vi "VITemplate.vi"(8 "Error In":errorcluster, 11 "Data In":T2) -> (0 "Error Out":errorcluster, 3 "Data Out":T2)   [LabVIEW 2019]
doc: "Description of VI"
uses:
  Controls/Data.ctl
  <vilib>/Utility/error.llb/DialogType.ctl
  <vilib>/Utility/miscctls.llb/LVPointTypeDef.ctl
panel:
  out "Control Tab":T1(tab)
  out "Console Out":string
  out "Error Message":string
  out "VI-filename":string
  out "Revision Number":u32
  out "VI Description":string
  out "Callers' Names":string[](array[string])
  out "Code Size":u32
  out "VI Type":T3(ring)
  out "Project name":string
  out "Project filepath":path
  out "VI filepath":path
  out "Project Description":string
  out "VI-Name":string
  # "Common Errors:"
  # "0:"
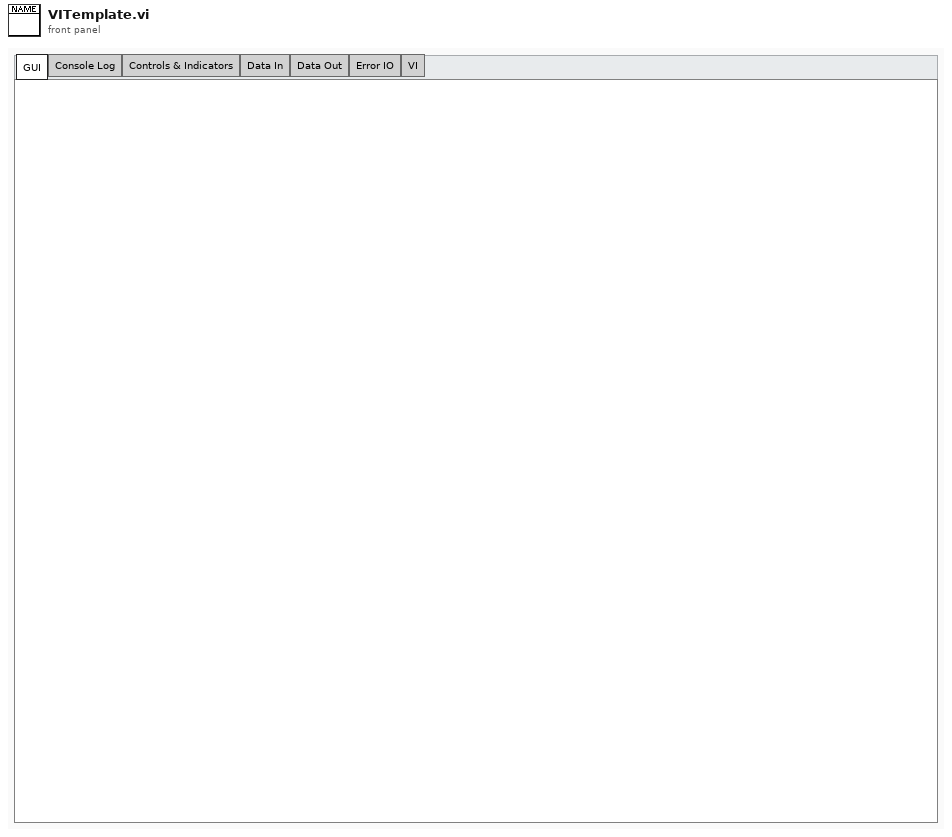
[diagram p1: front panel]
types:
  T1 = enum32{"GUI", "Console Log", "Controls & Indicators", "Data In", "Data Out", "Error IO", "VI"}
  T2 = typedef "Data.ctl" = cluster{"Log":string}
  T3 = enum32{"invalid VI type", "Standard VI", "Control VI", "Global VI", "Polymorphic VI", "Configuration VI", "SubSystem", "Facade VI", "Method VI", "Statechart Diagram VI"}
  T4 = typedef "LVPointTypeDef.ctl" = cluster{"Horizontal":i16, "Vertical":i16}
  T5 = typedef "DialogType.ctl" = u16
  T6 = typedef "LVRectTypeDef.ctl" = cluster{"Left":i16, "Top":i16, "Right":i16, "Bottom":i16}
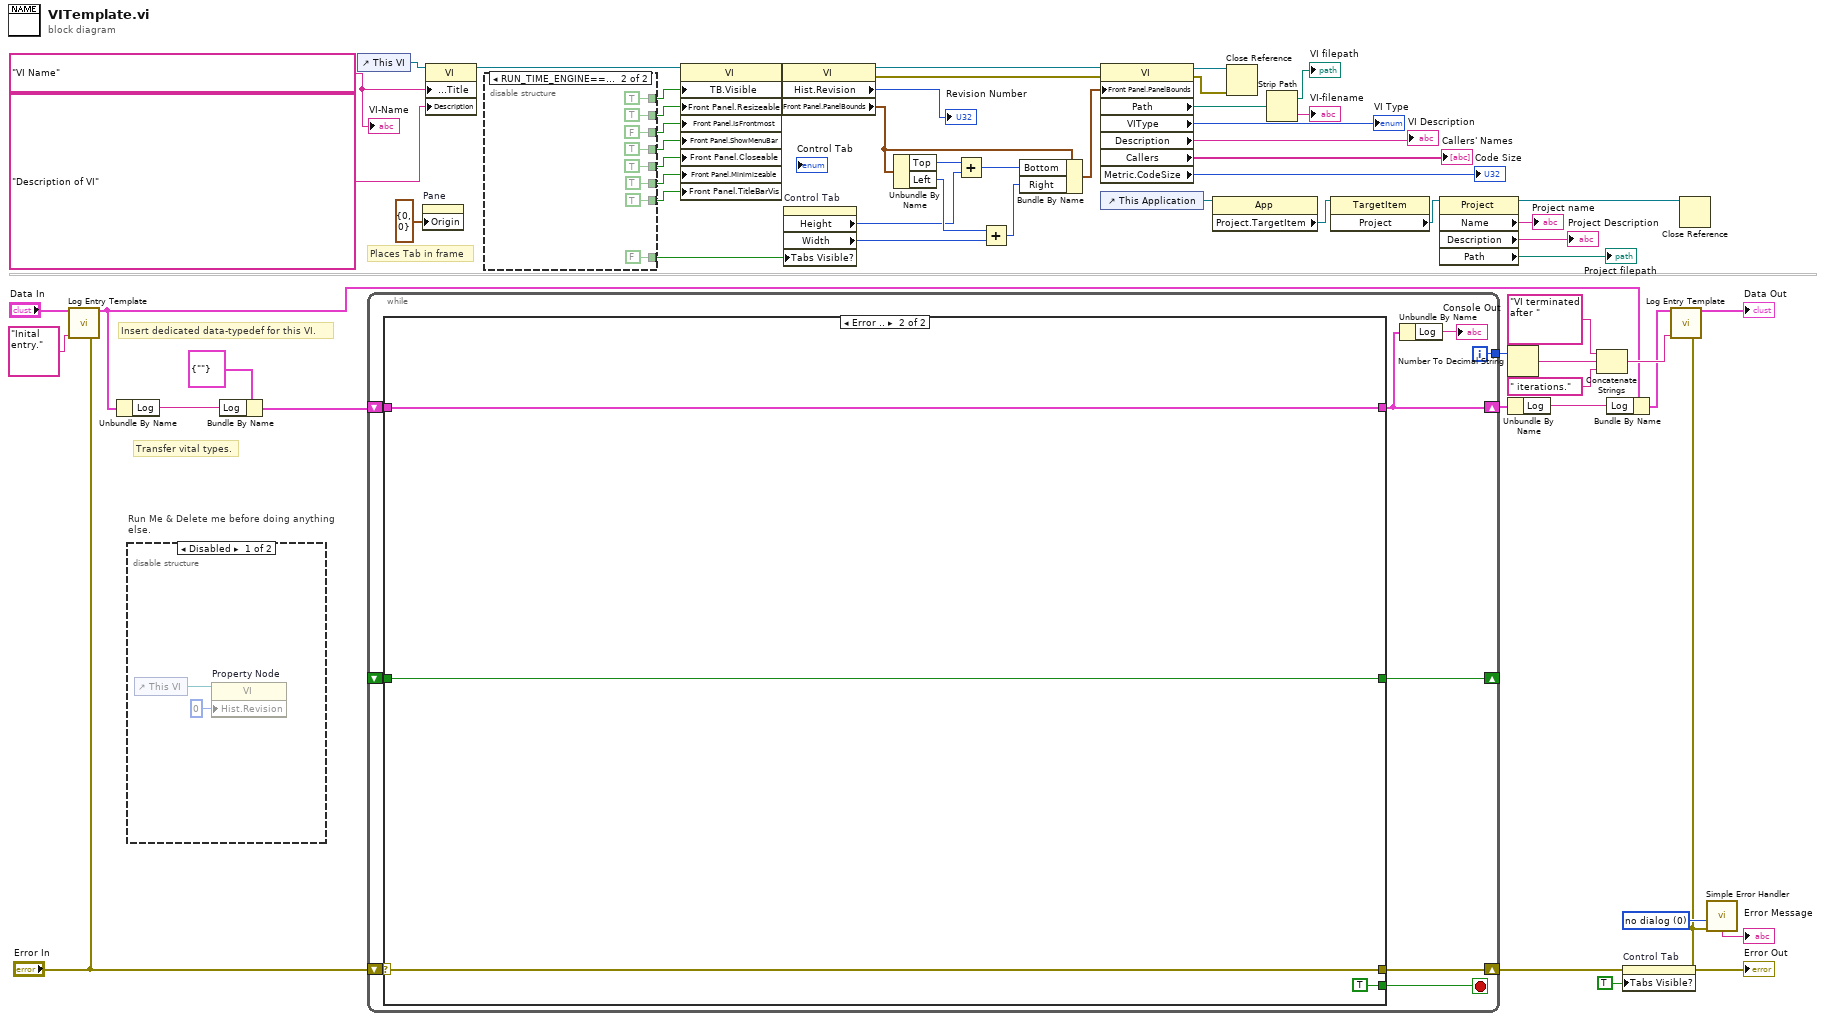
[diagram p0: block diagram]
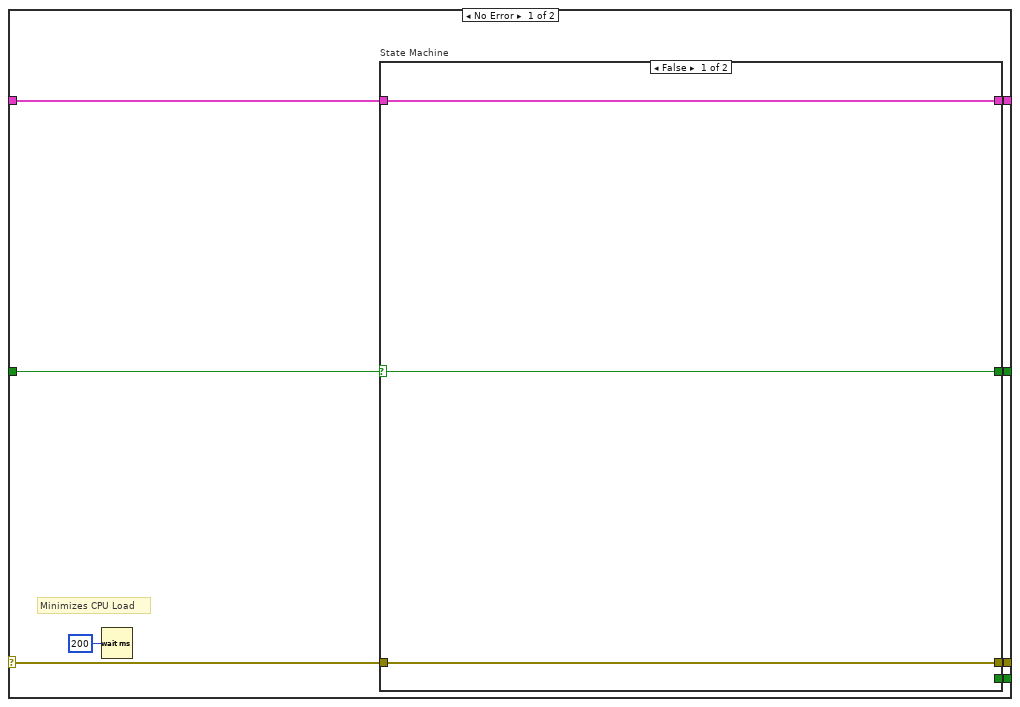
[diagram p2: hidden frame]
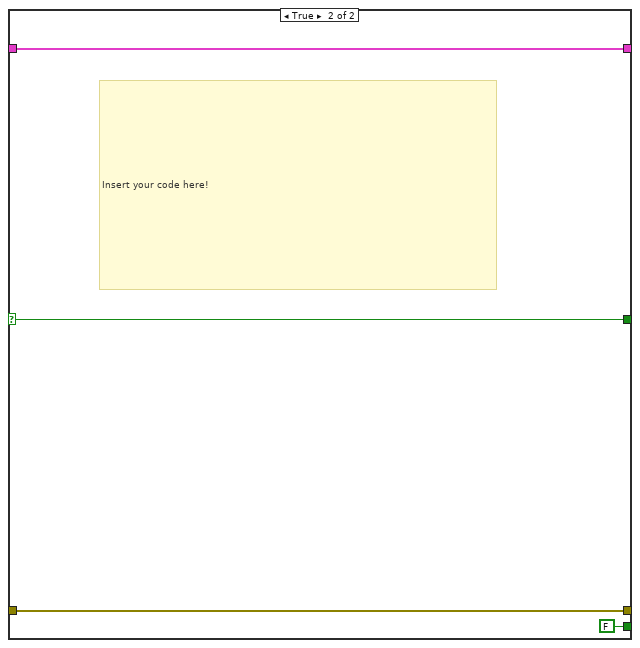
[diagram p3: hidden frame]
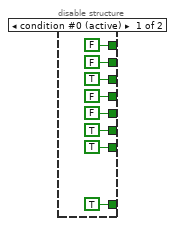
[diagram p5: hidden frame]
diagram:
  w32 = "VI Name"
  w60 = T5 0 items=["no dialog", "OK message", "continue or stop message", "OK message + warnings", "continue/stop + warnings"] ("type of dialog (OK msg:1)")
  # "Transfer vital types."
  # "Insert dedicated data-typedef for this VI."
  # "Places Tab in frame"
  n1 = call "Log Entry Template.vi"("Data In"="Data In", "Console Entry"="Inital entry.", "Error In"="Error In") -> ("Data Out"=w4:T2)  [unwired: 11 in, 1 out]
  n2 = Unbundle By Name(w4) -> ("Log"=w12:string)
  n3 = disable-structure "Run Me & Delete me before doing anything else." shown="Disabled" {
    frame Disabled {
      n4 = control-ref of="This VI"() -> (w65:refnum<vi>)
      n5 = property on="Property Node" class="VI"(reference=w65, "Hist.Revision"=u32 0 ("History:Revision Number")) -> ()  [unwired: 1 in, 2 out]
    }
    frame Enabled {
    }
  }
  n6 = Bundle By Name(cluster=T2 {"Log"=""} ("Data In"), "Log"=w12) -> (w11:T2)
  n7 = control-ref of="This VI"() -> (w44:refnum<vi>)
  n8 = while {
    shift-right: [w70] -> w14
    shift-left: "Error In" -> [w74]
    shift-right: [w72] -> _
    shift-left: _ -> [w71]
    shift-right: [w67] -> w5
    shift-left: w11 -> [w69]
    tunnel: [w68] -> w10
    i -> [w68]
    stop <- w73 stop-if-true
    n9 = case shown="Error .." w74 {
      selector: w74 -> [w79 w90]
      tunnel: [w82 TRUE] -> w73
      tunnel: [w81 w91] -> w72
      tunnel: w71 -> [w78 w91]
      tunnel: [w80 w90] -> w70
      tunnel: w69 -> [w77 w92]
      tunnel: [w76 w92] -> w67
      frame No Error {
        # "Minimizes CPU Load"
        n10 = Wait (ms)(milliseconds to wait=u32 200) -> ()  [unwired: 1 out]
        n11 = case "State Machine" shown="False" w78 {
          selector: w78 -> [w85 w88]
          tunnel: [_ FALSE] -> w82
          tunnel: [w85 w88] -> w81
          tunnel: [w83 w87] -> w80
          tunnel: w79 -> [w83 w87]
          tunnel: w77 -> [w84 w86]
          tunnel: [w84 w86] -> w76
          frame False {
          }
          frame True {
            # "Insert your code here!"
          }
        }
      }
      frame Error {
      }
    }
    n12 = Unbundle By Name(w67) -> ("Log"=→"Console Out":string)
  }
  n13 = property on="Pane" class="Pane"("Origin"=T4 {"Horizontal"=0, "Vertical"=0}) -> ()  [unwired: 2 in, 2 out]
  n14 = property class="VI"(reference=w44, "Front Panel.Title"=w32, "Description"="Description of VI") -> (reference out=w34:refnum<vi>)  [unwired: 1 in, 1 out]
  n15 = disable-structure "Exe vs Sim" shown="RUN_TIME_ENGINE==True" {
    disable-tunnel: [FALSE ("Tool Bar:Visible") TRUE ("Tool Bar:Visible")] -> w43
    disable-tunnel: [FALSE ("Front Panel Window:Resizable") TRUE ("Front Panel Window:Resizable")] -> w42
    disable-tunnel: [TRUE ("Front Panel Window:Is Frontmost") FALSE ("Front Panel Window:Is Frontmost")] -> w41
    disable-tunnel: [FALSE ("Front Panel Window:Show Menu Bar") TRUE ("Front Panel Window:Show Menu Bar")] -> w40
    disable-tunnel: [FALSE ("Front Panel Window:Closeable") TRUE ("Front Panel Window:Closeable")] -> w39
    disable-tunnel: [TRUE ("Front Panel Window:Title Bar Visible") TRUE ("Front Panel Window:Title Bar Visible")] -> w38
    disable-tunnel: [TRUE ("Front Panel Window:Minimizable") TRUE ("Front Panel Window:Minimizable")] -> w37
    disable-tunnel: [TRUE FALSE] -> w33
    frame condition #0 (active) {
    }
    frame condition #1 {
    }
  }
  n16 = property class="VI"(reference=w34, "TB.Visible"=w43, "Front Panel.Resizeable"=w42, "Front Panel.IsFrontmost"=w41, "Front Panel.ShowMenuBar"=w40, "Front Panel.Closeable"=w39, "Front Panel.Minimizeable"=w37, "Front Panel.TitleBarVis"=w38) -> (reference out=w36:refnum<vi>, error out=w35:errorcluster)  [unwired: 1 in]
  n17 = property class="VI"(reference=w36, error in=w35) -> (reference out=w50:refnum<vi>, error out=w46:errorcluster, "Hist.Revision"=→"Revision Number":u32, "Front Panel.PanelBounds"=w51:T6)
  n18 = property on="Control Tab" class="TabCtl (strict)"("Tabs Visible?"=w33) -> ("Height"=w53:u32, "Width"=w57:u32)  [unwired: 2 in, 2 out]
  n19 = Unbundle By Name(w51) -> ("Top"=w52:i16, "Left"=w56:i16)
  n20 = Add(x=w52, y=w53) -> (x+y=w54:u32)
  n21 = Add(x=w56, y=w57) -> (x+y=w55:u32)
  n22 = Bundle By Name(cluster=w51, "Bottom"=w54, "Right"=w55) -> (w49:T6)
  n23 = property on="Window size" class="VI"(reference=w50, error in=w46, "Front Panel.PanelBounds"=w49) -> (reference out=w58:refnum<vi>, error out=w47:errorcluster, "Path"=w31:path, "VIType"=→"VI Type":T3, "Description"=→"VI Description":string, "Callers"=→"Callers' Names":string[], "Metric.CodeSize"=→"Code Size":u32)
  n24 = control-ref of="This Application"() -> (w21:refnum<vi>)
  n25 = property class="App"(reference=w21) -> ("Project.TargetItem"=w26:refnum<vi>)  [unwired: 1 in, 2 out]
  n26 = Close Reference(reference=w58, error in (no error)=w47) -> ()  [unwired: 1 out]
  n27 = Strip Path(path=w31) -> (stripped path=→"VI filepath":path, name=→"VI-filename":string)
  n28 = property class="TargetItem"(reference=w26) -> ("Project"=w25:refnum<vi>)  [unwired: 1 in, 2 out]
  n29 = property class="Project"(reference=w25) -> (reference out=w19:refnum<vi>, "Name"=→"Project name":string, "Description"=→"Project Description":string, "Path"=→"Project filepath":path)  [unwired: 1 in, 1 out]
  n30 = Number To Decimal String(number=w10) -> (decimal integer string=w8:string)  [unwired: 1 in]
  n31 = Unbundle By Name(w5) -> ("Log"=w3:string)
  n32 = Concatenate Strings("VI terminated after " ("Console Entry"), w8, " iterations.") -> (w6:string)
  n33 = Bundle By Name(cluster=w4, "Log"=w3) -> (w2:T2)
  n34 = property on="Control Tab" class="TabCtl (strict)"(error in=w14, "Tabs Visible?"=TRUE) -> (error out=w15:errorcluster)  [unwired: 1 in, 1 out]
  "Error Out" <- w15
  n35 = call "Log Entry Template.vi"("Data In"=w2, "Console Entry"=w6, "Error In"=w15) -> ("Data Out"=→"Data Out":T2)  [unwired: 11 in, 1 out]
  n36 = Close Reference(reference=w19) -> ()  [unwired: 1 in, 1 out]
  n37 = call <vilib>:"Simple Error Handler.vi"("type of dialog (OK msg:1)"=w60, "error in (no error)"=w15) -> ("message"=→"Error Message":string)  [unwired: 3 in, 4 out]
  "VI-Name" <- w32
